vi "HostControl_Main_master.vi"() -> ()   [LabVIEW 2013]
uses:
  Messages.ctl
  PolarCoordTdef.ctl
  GainsTDef.ctl
  Support VIs/setpointCluster.ctl
  <vilib>/MakerHub/KinectOne/Private/Type Defs/Joint Position.ctl
  <vilib>/MakerHub/KinectOne/Private/Type Defs/JointType.ctl
  <vilib>/MakerHub/KinectOne/Private/Initialize Image [Color].vi
  <vilib>/MakerHub/KinectOne/Private/kinectRead [ColorFrame].vi
  <vilib>/MakerHub/KinectOne/Private/kinectRead [BodyFrame].vi
  Microsoft.Kinect
  C:/Program Files (x86)/National Instruments/LabVIEW 2013/vi.lib/MakerHub/KinectOne/Private/Libs/BodyFrameDataInterface.dll
  Program Files (x86)/National Instruments/LabVIEW 2013/vi.lib/MakerHub/KinectOne/Private/Libs/BodyFrameDataInterface.dll
  <vilib>/MakerHub/KinectOne/KinectOne.lvlib
panel:
  in  "Kd-Argument":dbl
  in  "Kc-Argument":dbl
  in  "Kd-Modulus":dbl
  in  "Kc-Modulus":dbl
  in  "Argument Setpoint":dbl
  in  "Modulus Setpoint":dbl=1.8
  out "Image":T1(plugin-control)
  out "Mod":dbl
  out "Arg":dbl
  in  "IT'S TIME TO":bool
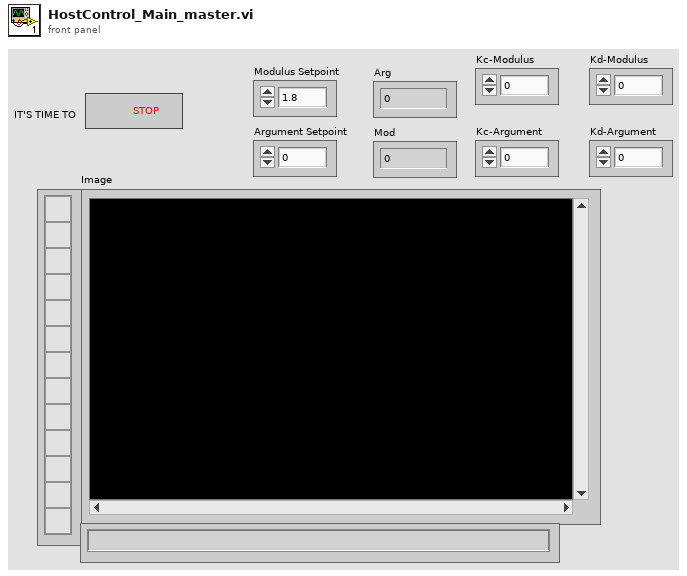
[diagram p1: front panel]
types:
  T1 = typedef "IMAQ Image.ctl" = refnum<image>
  T2 = typedef "Messages.ctl" = cluster{"message data":variant, "message type":enum16{"Stop", "PolarCoordinates", "Gains", "Setpoints"}}
  T3 = typedef "KinectOne.lvlib/KinectSensor References.ctl" = cluster{"KinectSensor":refnum<k24>, "MultiSourceFrameReader":refnum<k24>, "BodyFrameDataInterface":refnum<k24>}
  T4 = enum16{"Stop", "PolarCoordinates", "Gains", "Setpoints"}
  T5 = typedef "PolarCoordTdef.ctl" = cluster{"Argument":dbl, "Modulus":dbl}
  T6 = typedef "KinectOne.lvlib/Joint Position.ctl" = cluster{"Camera Space":cluster{"X":dbl, "Y":dbl, "Z":dbl}, "Color Space":cluster{"X":dbl, "Y":dbl}, "Depth Space":cluster{"X":dbl, "Y":dbl}, "Tracking State":enum16{"NotTracked", "Inferred", "Tracked"}}
  T7 = typedef "KinectOne.lvlib/JointType.ctl" = enum16{"SpineBase", "SpineMid", "Neck", "Head", "ShoulderLeft", "ElbowLeft", "WristLeft", "HandLeft", "ShoulderRight", "ElbowRight", "WristRight", "HandRight", "HipLeft", "KneeLeft", "AnkleLeft", "FootLeft", "HipRight", "KneeRight", "AnkleRight", "FootRight", "SpineShoulder", "HandTipLeft", "ThumbLeft", "HandTipRight", "ThumbRight"}
  T8 = typedef "KinectOne.lvlib/BodyData.ctl" = cluster{"ClippedEdges":T9, "HandLeftConfidence":T10, "HandLeftState":T11, "HandRightConfidence":T12, "HandRightState":T13, "IsRestricted":bool, "IsTracked":bool, "JointOrientations":refnum<k24>, "Joints":refnum<k24>, "Lean":refnum<k24>, "LeanTrackingState":T14, "TrackingId":u64}
  T9 = typedef "KinectOne.lvlib/ClippedEdges.ctl" = enum16{"None", "Right", "Left", "Top", "Bottom"}
  T10 = typedef "KinectOne.lvlib/HandLeftConfidence.ctl" = enum16{"Low", "High"}
  T11 = typedef "KinectOne.lvlib/HandLeftState.ctl" = enum16{"Unknown", "NotTracked", "Open", "Closed", "Lasso"}
  T12 = typedef "KinectOne.lvlib/HandRightConfidence.ctl" = enum16{"Low", "High"}
  T13 = typedef "KinectOne.lvlib/HandRightState.ctl" = enum16{"Unknown", "NotTracked", "Open", "Closed", "Lasso"}
  T14 = typedef "KinectOne.lvlib/LeanTrackingState.ctl" = enum16{"NotTracked", "Inferred", "Tracked"}
  T15 = typedef "setpointCluster.ctl" = cluster{"Modulus Setpoint":dbl, "Argument Setpoint":dbl}
  T16 = typedef "GainsTDef.ctl" = cluster{"Kc-Modulus":dbl, "Kd-Argument":dbl, "Kd-Modulus":dbl, "Kc-Argument":dbl}
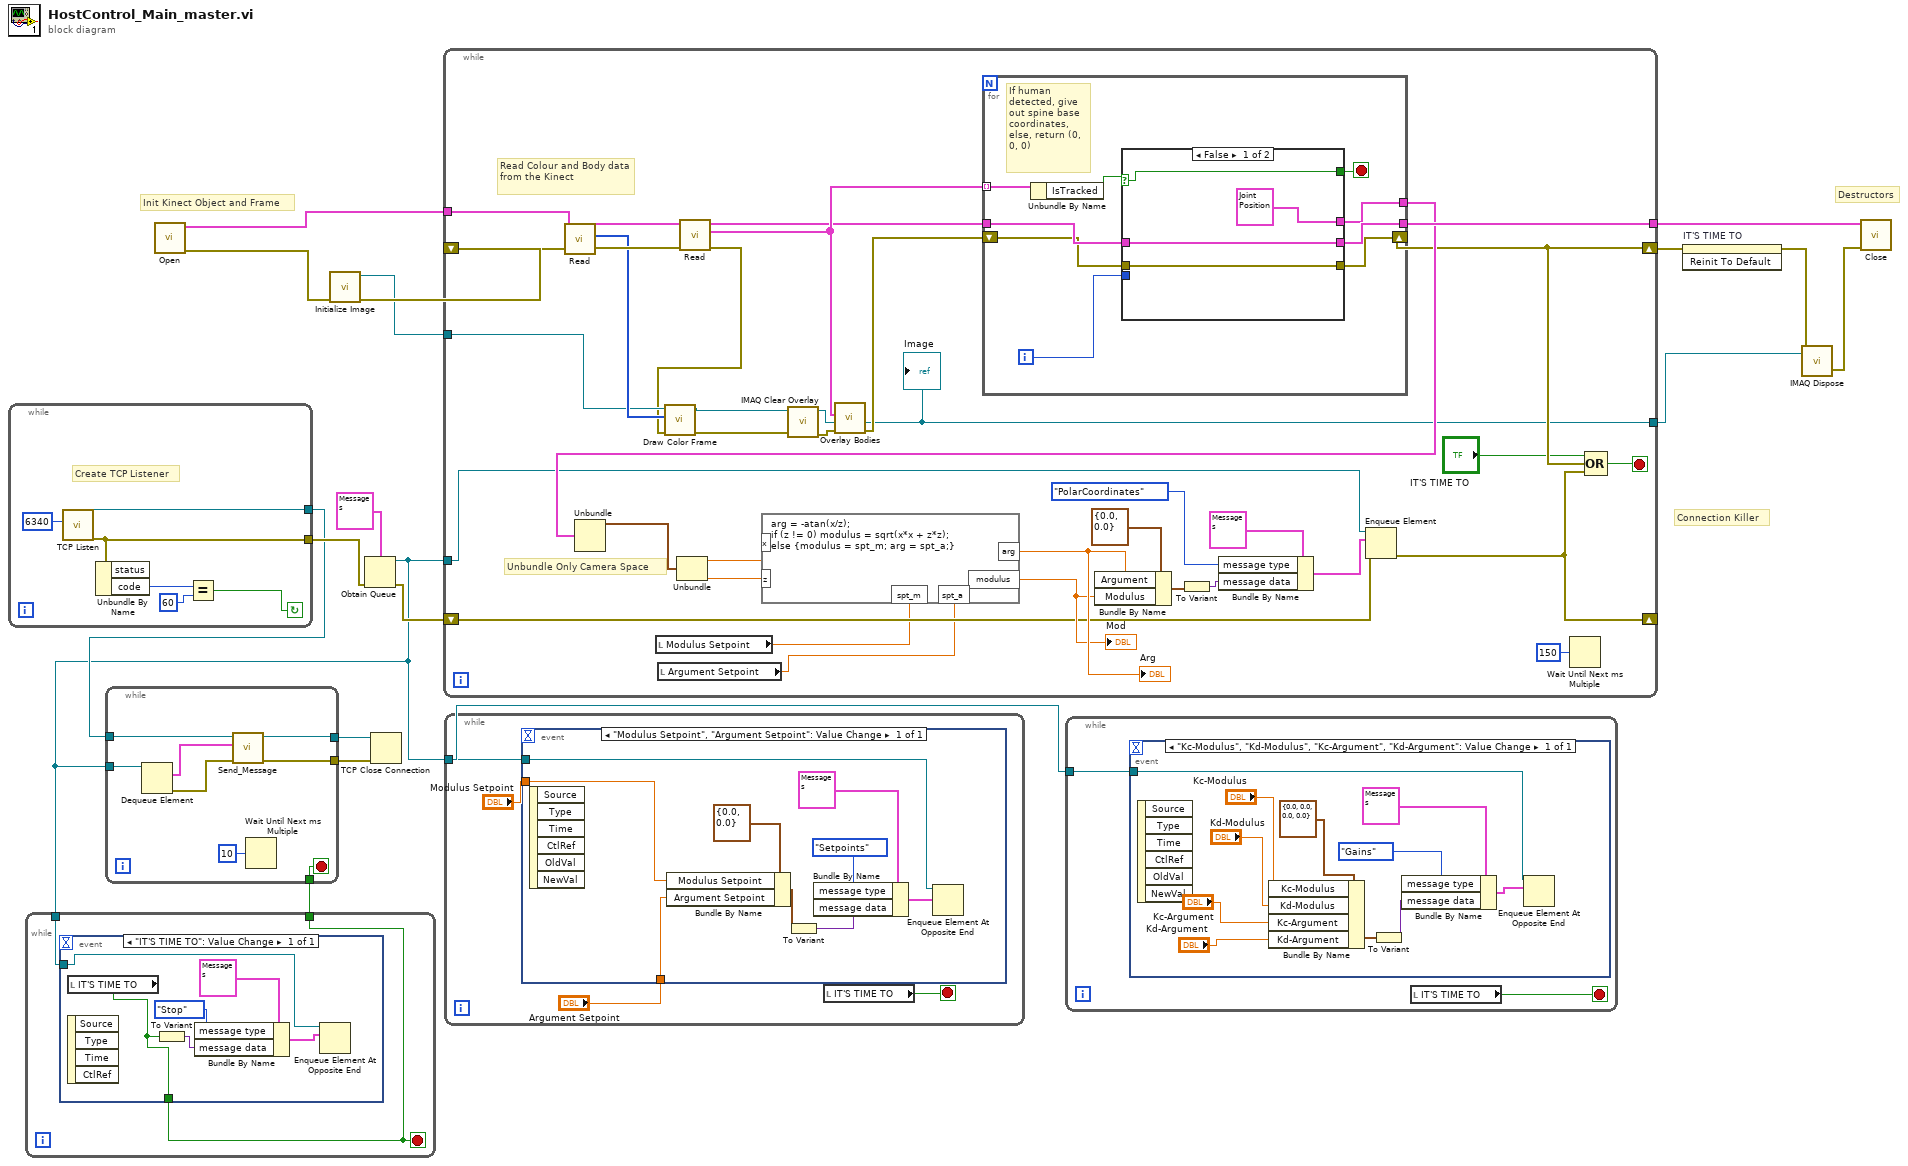
[diagram p0: block diagram]
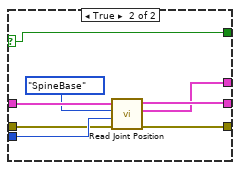
[diagram p2: hidden frame]
diagram:
  # "Connection Killer"
  # "Destructors"
  # "Init Kinect Object and Frame"
  n1 = while {
    tunnel: [w22] -> w7
    tunnel: [w21] -> w10
    stop <- w18 continue-if-true
    # "Create TCP Listener"
    n2 = call <vilib>:"TCP Listen.vi"("port"=u16 6340) -> ("error out"=w21:errorcluster, "connection ID"=w22:refnum<k5>)  [unwired: 6 in, 3 out]
    n3 = Unbundle By Name(w21) -> ("code"=w20:i32)  [unwired: 1 out]
    n4 = Equal?(x=w20, y=60) -> (x = y?=w18:bool)
  }
  n5 = call <vilib>:"Open.vi"() -> ("Error Out"=w16:errorcluster, "KinectSensor References out"=w17:T3)  [unwired: 10 in]
  n6 = call-poly <vilib>:"Initialize Image.vi"("Error In"=w16) -> ("Error Out"=w15:errorcluster, "Color Image"=w14:T1)  [unwired: 9 in]
  n7 = Obtain Queue(element data type=T2 {"message data"=variant, "message type"=enum."Stop"} ("message"), error in (no error)=w10) -> (queue out=w4:refnum<queue>, error out=w9:errorcluster)  [unwired: 3 in, 1 out]
  n8 = while {
    tunnel: w4 -> [w25]
    tunnel: [w24] -> w3
    stop <- w24 stop-if-true
    n9 = event shown="[0] \"IT'S TIME TO\": Value Change" {
      selector: _ -> [_]
      dyn-events: _ -> [_]
      timeout: _ -> [_]
      tunnel: [w27] -> w24
      tunnel: w25 -> [w29]
      event "IT'S TIME TO": Value Change {
        n10 = local read "IT'S TIME TO"() -> (w27:bool)
        n11 = event-data() -> ()  [unwired: 1 in, 4 out]
        n12 = To Variant(anything=w27) -> (Variant=w28:variant)
        n13 = Bundle By Name(cluster=T2 {"message data"=variant, "message type"=enum."Stop"} ("message"), "message type"=T4."Stop", "message data"=w28) -> (w26:T2)
        n14 = Enqueue Element At Opposite End(queue=w29, element=w26) -> ()  [unwired: 2 in, 3 out]
      }
    }
  }
  n15 = while {
    tunnel: w7 -> [w39]
    tunnel: w4 -> [w38]
    tunnel: [w34] -> w6
    tunnel: [w33] -> w5
    tunnel: w3 -> [w32]
    stop <- w32 stop-if-true
    n16 = Dequeue Element(queue=w38) -> (element=w37:T2, error out=w36:errorcluster)  [unwired: 2 in, 2 out]
    n17 = call "Send_Message.vi"("error in (no error)"=w36, "message"=w37, "connection ID"=w39) -> ("error out (no error)"=w33:errorcluster, "connection ID 2"=w34:refnum<k5>)  [unwired: 7 in]
    n18 = Wait Until Next ms Multiple(millisecond multiple=u32 10 ("milliseconds to wait")) -> ()  [unwired: 1 out]
  }
  n19 = TCP Close Connection(connection ID=w6, error in (no error)=w5) -> ()  [unwired: 1 in, 2 out]
  n20 = while {
    tunnel: w17 -> [w55]
    tunnel: w14 -> [w51]
    shift-right: [w67] -> w2
    shift-left: w15 -> [w57]
    tunnel: [w72] -> w13
    shift-right: [w43] -> _
    shift-left: w9 -> [w44]
    tunnel: [w47] -> w11
    tunnel: w4 -> [w42]
    stop <- w61 stop-if-true
    # "Unbundle Only Camera Space"
    # "Read Colour and Body data from the Kinect"
    n21 = call-poly <vilib>:"Read.vi"("Error In"=w57, "KinectSensor References in"=w55) -> ("Error Out"=w56:errorcluster, "frameData"=w52:u32[], "KinectSensor References out"=w54:T3)  [unwired: 7 in]
    n22 = local read "Modulus Setpoint"() -> (w41:dbl)
    n23 = local read "Argument Setpoint"() -> (w40:dbl)
    n24 = call-poly <vilib>:"Read.vi"("error in (no error)"=w56, "KinectSensor References in"=w54) -> ("error out"=w49:errorcluster, "Body Data"=w74:T8[], "KinectSensor References out"=w73:T3)  [unwired: 7 in]
    n25 = call <vilib>:"Draw Color Frame.vi"("Error In"=w49, "U32 Array"=w52, "Image"=w51) -> ("Error Out"=w48:errorcluster, "Image Out"=w50:T1)  [unwired: 7 in]
    n26 = call "IMAQ Clear Overlay"("error in (no error)"=w48, "Image"=w50) -> ("error out"=w76:errorcluster, "Image Out"=w75:T1)  [unwired: 8 in]
    n27 = call <vilib>:"Overlay Bodies.vi"("Error In"=w76, "Image"=w75, "Body Data"=w74) -> ("Error Out"=w53:errorcluster, "Image Out"=w47:T1)  [unwired: 7 in]
    "Image" <- w47
    n28 = for {
      shift-right: [w79] -> w67
      shift-left: w53 -> [w80]
      tunnel: w74 -> [w85] mode=indexing
      tunnel: w73 -> [w84]
      tunnel: [w83] -> w72
      tunnel: [w81] -> w71
      i -> [w82]
      stop <- w77 stop-if-true
      # "If human detected, give out spine base coordinates,\nelse, return (0, 0, 0)"
      n29 = Unbundle By Name(w85) -> ("IsTracked"=w78:bool)
      n30 = case shown="False" w78 {
        selector: w78 -> [w86 w92]
        tunnel: w84 -> [w89 w97]
        tunnel: [w89 w96] -> w83
        tunnel: w82 -> [_ w94]
        tunnel: [T6 {"Camera Space"={"X"=0.0, "Y"=0.0, "Z"=0.0}, "Color Space"={"X"=0.0, "Y"=0.0}, "Depth Space"={"X"=0.0, "Y"=0.0}, "Tracking State"=enum."NotTracked"} ("Joint Position") w93] -> w81
        tunnel: w80 -> [w87 w91]
        tunnel: [w87 w90] -> w79
        tunnel: [w86 w92] -> w77
        frame False {
        }
        frame True {
          n31 = call <vilib>:"Read Joint Position.vi"("Error In"=w91, "Body Index"=w94, "JointType"=JointType."SpineBase", "KinectSensor References"=w97) -> ("Error Out"=w90:errorcluster, "Joint Position"=w93:T6, "KinectSensor References"=w96:T3)  [unwired: 4 in, 1 out]
        }
      }
    }
    n32 = Unbundle(w71) -> ("Camera Space"=w70:cluster{"X":dbl, "Y":dbl, "Z":dbl})  [unwired: 3 out]
    n33 = Unbundle(w70) -> ("X"=w64:dbl, "Z"=w63:dbl)  [unwired: 1 out]
    n34 = formula code="arg = -atan(x/z);\nif (z != 0) modulus = sqrt(x*x + z*z);\nelse {modulus = spt_m; arg = spt_a;}"("x"=w64, "z"=w63, "spt_m"=w41, "spt_a"=w40) -> ("arg"=w60:dbl, "modulus"=w59:dbl)
    "Arg" <- w60
    "Mod" <- w59
    n35 = Bundle By Name(cluster=T5 {"Argument"=0.0, "Modulus"=0.0}, "Argument"=w60, "Modulus"=w59) -> (w65:T5)
    n36 = To Variant(anything=w65) -> (Variant=w66:variant)
    n37 = Bundle By Name(cluster=T2 {"message data"=variant, "message type"=enum."Stop"} ("message"), "message type"=T4."PolarCoordinates", "message data"=w66) -> (w45:T2)
    n38 = Enqueue Element(queue=w42, element=w45, error in (no error)=w44) -> (error out=w43:errorcluster)  [unwired: 1 in, 2 out]
    n39 = Wait Until Next ms Multiple(millisecond multiple=u32 150) -> ()  [unwired: 1 out]
    n40 = Compound Arithmetic op=OR("IT'S TIME TO", w67, w43) -> (w61:bool)
  }
  n41 = while {
    tunnel: w4 -> [w101]
    stop <- w100 stop-if-true
    n42 = event shown="[0] \"Modulus Setpoint\", \"Argument Setpoint\": Value Change" {
      selector: _ -> [_]
      dyn-events: _ -> [_]
      timeout: _ -> [_]
      tunnel: w101 -> [w105]
      tunnel: "Argument Setpoint" -> [w103]
      tunnel: "Modulus Setpoint" -> [w102]
      event "Modulus Setpoint", "Argument Setpoint": Value Change {
        n43 = event-data() -> ()  [unwired: 1 in, 6 out]
        n44 = Bundle By Name(cluster=T15 {"Modulus Setpoint"=0.0, "Argument Setpoint"=0.0} ("Setpoint Cluster"), "Modulus Setpoint"=w102, "Argument Setpoint"=w103) -> (w104:T15)
        n45 = To Variant(anything=w104) -> (Variant=w107:variant)
        n46 = Bundle By Name(cluster=T2 {"message data"=variant, "message type"=enum."Stop"} ("message"), "message type"=T4."Setpoints", "message data"=w107) -> (w106:T2)
        n47 = Enqueue Element At Opposite End(queue=w105, element=w106) -> ()  [unwired: 2 in, 3 out]
      }
    }
    n48 = local read "IT'S TIME TO"() -> (w100:bool)
  }
  n49 = while {
    tunnel: w4 -> [w112]
    stop <- w111 stop-if-true
    n50 = event shown="[0] \"Kc-Modulus\", \"Kd-Modulus\", \"Kc-Argument\", \"Kd-Argument\": Value Change" {
      selector: _ -> [_]
      dyn-events: _ -> [_]
      timeout: _ -> [_]
      tunnel: w112 -> [w113]
      event "Kc-Modulus", "Kd-Modulus", "Kc-Argument", "Kd-Argument": Value Change {
        n51 = event-data() -> ()  [unwired: 1 in, 6 out]
        n52 = Bundle By Name(cluster=T16 {"Kc-Modulus"=0.0, "Kd-Argument"=0.0, "Kd-Modulus"=0.0, "Kc-Argument"=0.0}, "Kc-Modulus"="Kc-Modulus", "Kd-Modulus"="Kd-Modulus", "Kc-Argument"="Kc-Argument", "Kd-Argument"="Kd-Argument") -> (w118:T16)
        n53 = To Variant(anything=w118) -> (Variant=w117:variant)
        n54 = Bundle By Name(cluster=T2 {"message data"=variant, "message type"=enum."Stop"} ("message"), "message type"=T4."Gains", "message data"=w117) -> (w114:T2)
        n55 = Enqueue Element At Opposite End(queue=w113, element=w114) -> ()  [unwired: 2 in, 3 out]
      }
    }
    n56 = local read "IT'S TIME TO"() -> (w111:bool)
  }
  n57 = invoke on="IT'S TIME TO" class="Bool (strict)" method="Reinit To Default"(error in=w2) -> (error out=w1:errorcluster)  [unwired: 2 in, 2 out]
  n58 = call "IMAQ Dispose"("Image"=w11, "error in (no error)"=w1) -> ("error out"=w12:errorcluster)  [unwired: 4 in]
  n59 = call <vilib>:"Close.vi"("Error In"=w12, "KinectSensor References"=w13) -> ()  [unwired: 9 in, 1 out]
